vi "Close.vi"(8 "error in (no error)":errorcluster, 11 "PowerSupply_IT6333A in":refnum<class "PowerSupply_IT6333A.lvclass">) -> (0 "error out":errorcluster, 3 "PowerSupply_IT6333A out":refnum<class "PowerSupply_IT6333A.lvclass">)   [LabVIEW 2013, in "PowerSupply_IT6333A.lvclass"]
uses:
  PowerSupply_IT6333A.lvclass
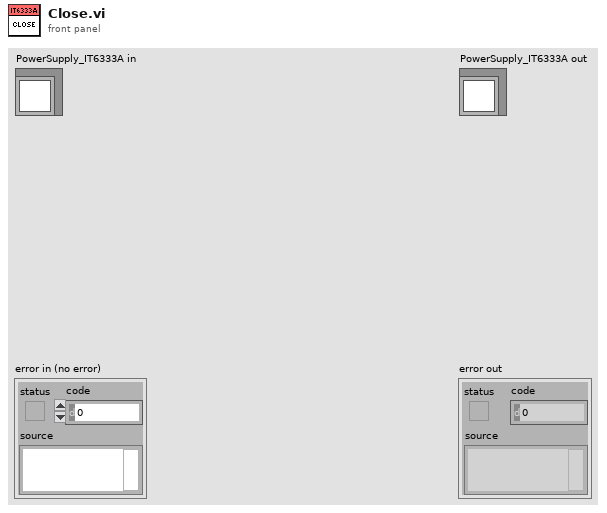
[diagram p1: front panel]
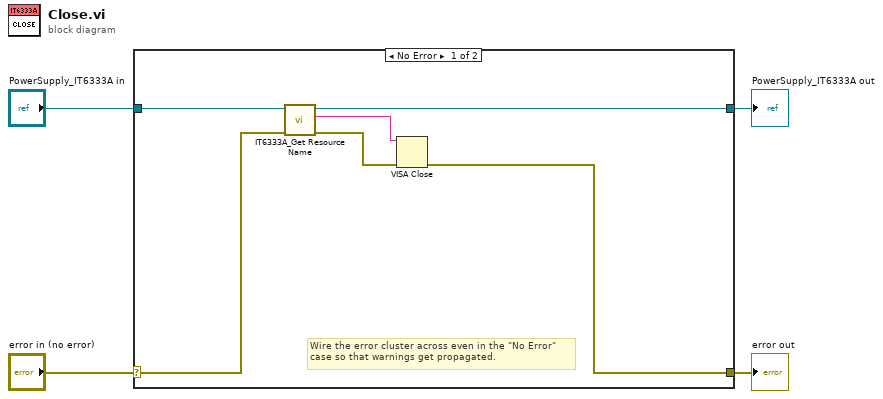
[diagram p0: block diagram]
diagram:
  n1 = case shown="No Error" "error in (no error)" {
    selector: "error in (no error)" -> [w6 w12]
    tunnel: [w5 w12] -> w3
    tunnel: [w9 w11] -> w1
    tunnel: "PowerSupply_IT6333A in" -> [w10 w11]
    frame No Error {
      # "Wire the error cluster across even in the \"No Error\"\ncase so that warnings get propagated."
      n2 = call-dynamic "IT6333A_Get Resource Name.vi"("error in (no error)"=w6, "PowerSupply_IT6333A in"=w10) -> ("error out"=w7:errorcluster, "Resource Name"=w8:string, "PowerSupply_IT6333A out"=w9:refnum<class "PowerSupply_IT6333A.lvclass">)  [unwired: 7 in]
      n3 = VISA Close(VISA resource name=w8, error in (no error)=w7) -> (error out=w5:errorcluster)
    }
    frame Error {
    }
  }
  "error out" <- w3
  "PowerSupply_IT6333A out" <- w1
